vi "Trim Pulse Data for Shift.vi"(8 "error in (no error)":errorcluster, 10 "date time rec":T1, 11 "Parsed Pulse Data":T2(array[cluster])) -> (0 "error out":errorcluster, 2 "Shift Start Time":T1, 3 "Shift Pulse Data":T2(array[cluster]))   [LabVIEW 2013, in "Controls Log Monitor.lvlib"]
uses:
  <vilib>/Utility/miscctls.llb/LVDateTimeRec.ctl
  Controls Log Monitor.lvlib
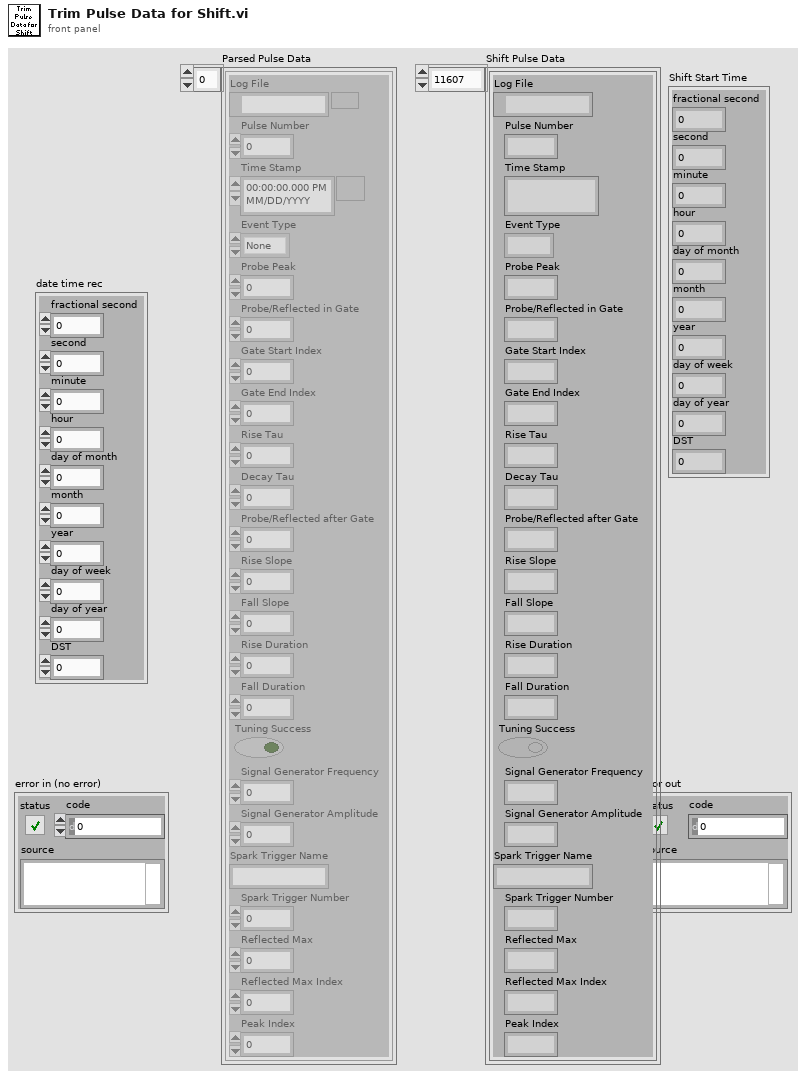
[diagram p1: front panel]
types:
  T1 = typedef "LVDateTimeRec.ctl" = cluster{"fractional second":dbl, "second":i32, "minute":i32, "hour":i32, "day of month":i32, "month":i32, "year":i32, "day of week":i32, "day of year":i32, "DST":i32}
  T2 = cluster{"Log File":path, "Pulse Number":u32, "Time Stamp":timestamp, "Event Type":enum16{"None", "Tune", "Periodic Capture", "Spark Trigger"}, "Probe Peak":dbl, "Probe/Reflected in Gate":dbl, "Gate Start Index":i32, "Gate End Index":i32, "Rise Tau":dbl, "Decay Tau":dbl, "Probe/Reflected after Gate":dbl, "Rise Slope":dbl, "Fall Slope":dbl, "Rise Duration":dbl, "Fall Duration":dbl, "Tuning Success":bool, "Signal Generator Frequency":dbl, "Signal Generator Amplitude":dbl, "Spark Trigger Name":string, "Spark Trigger Number":i32, "Reflected Max":dbl, "Reflected Max Index":i32, "Peak Index":i32}[]
  T3 = cluster{"Log File":path, "Pulse Number":u32, "Time Stamp":timestamp, "Event Type":enum16{"None", "Tune", "Periodic Capture", "Spark Trigger"}, "Probe Peak":dbl, "Probe/Reflected in Gate":dbl, "Gate Start Index":i32, "Gate End Index":i32, "Rise Tau":dbl, "Decay Tau":dbl, "Probe/Reflected after Gate":dbl, "Rise Slope":dbl, "Fall Slope":dbl, "Rise Duration":dbl, "Fall Duration":dbl, "Tuning Success":bool, "Signal Generator Frequency":dbl, "Signal Generator Amplitude":dbl, "Spark Trigger Name":string, "Spark Trigger Number":i32, "Reflected Max":dbl, "Reflected Max Index":i32, "Peak Index":i32}
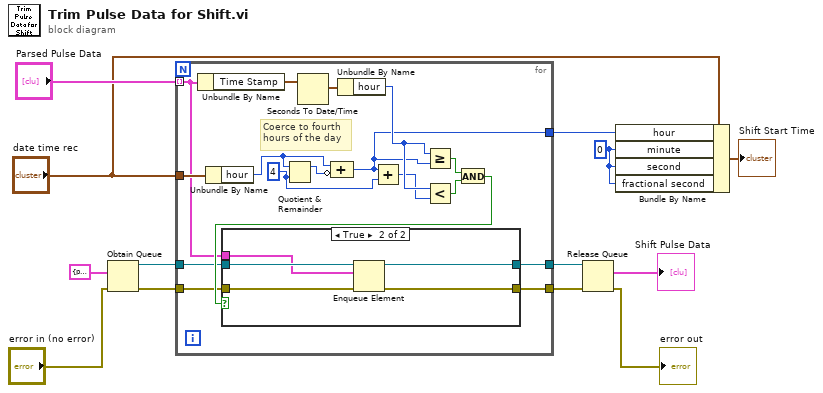
[diagram p0: block diagram]
diagram:
  w3 = 0 ("minute")
  n1 = Obtain Queue(element data type=T3 {"Log File"=path "", "Pulse Number"=0, "Time Stamp"=timestamp(0 s since 1904-01-01), "Event Type"=enum."None", "Probe Peak"=0.0, "Probe/Reflected in Gate"=0.0, "Gate Start Index"=0, "Gate End Index"=0, "Rise Tau"=0.0, "Decay Tau"=0.0, "Probe/Reflected after Gate"=0.0, "Rise Slope"=0.0, "Fall Slope"=0.0, "Rise Duration"=0.0, "Fall Duration"=0.0, "Tuning Success"=FALSE, "Signal Generator Frequency"=0.0, "Signal Generator Amplitude"=0.0, "Spark Trigger Name"="", "Spark Trigger Number"=0, "Reflected Max"=0.0, "Reflected Max Index"=0, "Peak Index"=0} ("Pulse Data Cluster"), error in (no error)="error in (no error)") -> (queue out=w10:refnum<queue>, error out=w6:errorcluster)  [unwired: 3 in, 1 out]
  n2 = for {
    tunnel: "Parsed Pulse Data" -> [w22] mode=indexing
    tunnel: "date time rec" -> [w28]
    tunnel: w10 -> [w24]
    tunnel: [w23] -> w9
    tunnel: w6 -> [w21]
    tunnel: [w20] -> w5
    tunnel: [w16] -> w4
    w15 = 4 ("y")
    # "Coerce to fourth\nhours of the day"
    n3 = Unbundle By Name(w22) -> ("Time Stamp"=w30:timestamp)
    n4 = Unbundle By Name(w28) -> ("hour"=w18:i32)
    n5 = Quotient & Remainder(x=w18, y=w15) -> (x-y*floor(x/y)=w17:i32)  [unwired: 1 out]
    n6 = Seconds To Date/Time(time stamp (now)=w30) -> (date time rec=w29:T1)  [unwired: 1 in]
    n7 = Compound Arithmetic op=unknown(w18, invert w17) -> (w16:i32)
    n8 = Unbundle By Name(w29) -> ("hour"=w19:i32)
    n9 = Add(x=w16, y=w15) -> (x+y=w14:i32)
    n10 = Greater Or Equal?(x=w19, y=w16) -> (x >= y?=w26:bool)
    n11 = Less?(x=w19, y=w14) -> (x < y?=w27:bool)
    n12 = And(x=w26, y=w27) -> (x .and. y?=w25:bool)
    n13 = case shown="True" w25 {
      tunnel: w24 -> [w32 w37]
      tunnel: [w32 w36] -> w23
      tunnel: w22 -> [_ w35]
      tunnel: w21 -> [w31 w34]
      tunnel: [w31 w33] -> w20
      frame False {
      }
      frame True {
        n14 = Enqueue Element(queue=w37, element=w35, error in (no error)=w34) -> (queue out=w36:refnum<queue>, error out=w33:errorcluster)  [unwired: 1 in, 1 out]
      }
    }
  }
  n15 = Release Queue(queue=w9, error in (no error)=w5) -> (remaining elements=→"Shift Pulse Data":T2, error out=→"error out":errorcluster)  [unwired: 1 in, 1 out]
  n16 = Bundle By Name(cluster="date time rec", "hour"=w4, "minute"=w3, "second"=w3, "fractional second"=w3) -> (→"Shift Start Time":T1)
